vi "Write Collider.vi"(8 "error in (no error)":errorcluster, 10 "Collider in":refnum<class "Collider.lvclass">, 11 "SimulationObject in":refnum<class "SimulationObject.lvclass">) -> (0 "error out":errorcluster, 3 "SimulationObject out":refnum<class "SimulationObject.lvclass">)   [LabVIEW 2022 SP3, in "SimulationObject.lvclass"]
uses:
  SimulationObject.lvclass
  Collisions/Collider/Collider.lvclass
  SimulationObject.lvclass/SimulationObject.ctl
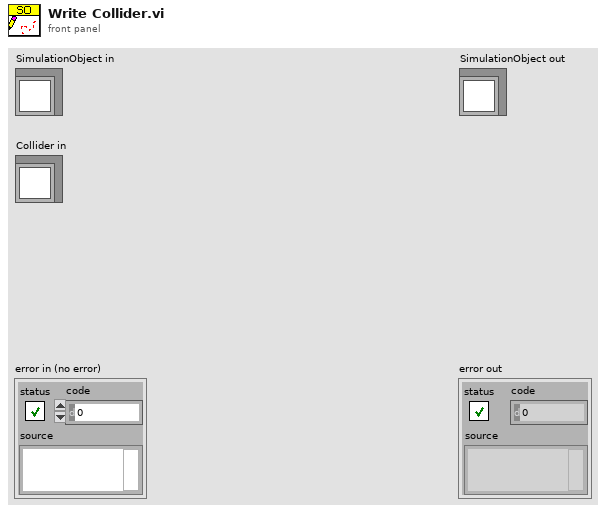
[diagram p1: front panel]
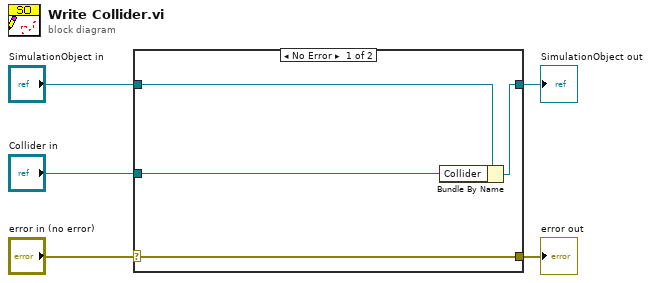
[diagram p0: block diagram]
diagram:
  n1 = case shown="No Error" "error in (no error)" {
    selector: "error in (no error)" -> [w9 w10]
    tunnel: [w9 w10] -> w4
    tunnel: [w7 w11] -> w2
    tunnel: "SimulationObject in" -> [w8 w11]
    tunnel: "Collider in" -> [w6 _]
    frame No Error {
      n2 = Bundle By Name(cluster=w8, "Collider"=w6) -> (w7:refnum<class "SimulationObject.lvclass">)
    }
    frame Error {
    }
  }
  "error out" <- w4
  "SimulationObject out" <- w2
